vi "Process XML Node old2.vi"(8 "Error in":errorcluster caption="Error in (no error)", 11 "XML Element":refnum<k20>) -> (0 "Error out":errorcluster, 1 "Is Array?":bool, 2 "Attribute":refnum<class "Attribute.lvclass">, 3 "XML Element Out":refnum<k20>)   [LabVIEW 2018]
uses:
  Attribute.lvclass
  Data Item.lvclass/Data Item.ctl
  Element.lvclass/Element.ctl
  Element.lvclass
  C:/Users/Flarn/Documents/LabVIEW Projects/Low-Level VI Manipulation/Support Files/VILab/Data Item.lvclass
  Attribute.lvclass/Attribute.ctl
  Attribute/Create Attribute (Data Item).vi
  Element Array.lvclass
  Data Item.lvclass
  <vilib>/xml/NI_XML.lvlib
  <resource>/objmgr/DOMUserDefRef.rc
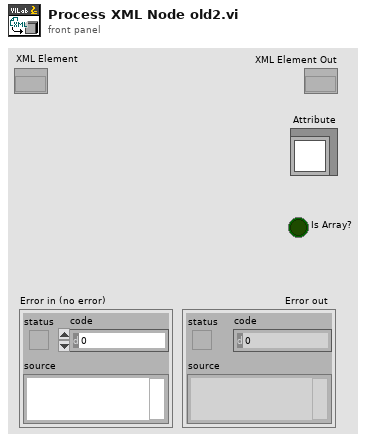
[diagram p1: front panel]
types:
  T1 = cluster{"class":string, "uid":string, "Attributes":refnum<class "Attribute.lvclass">[], "Array?":bool}
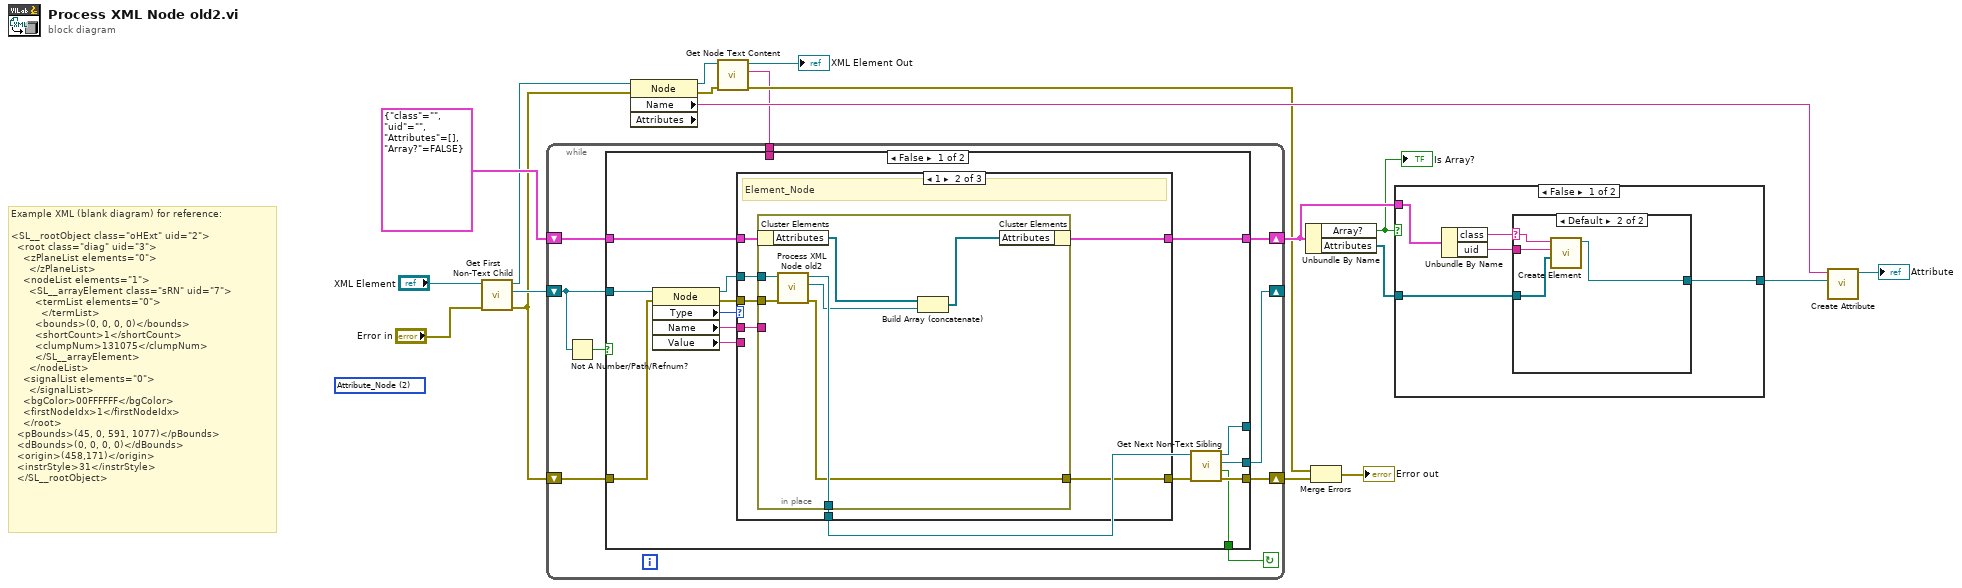
[diagram p0: block diagram]
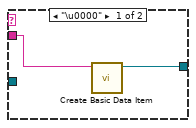
[diagram p2: hidden frame]
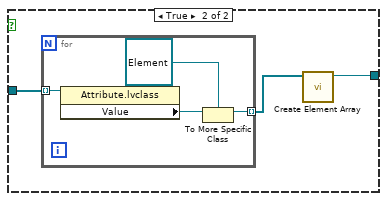
[diagram p3: hidden frame]
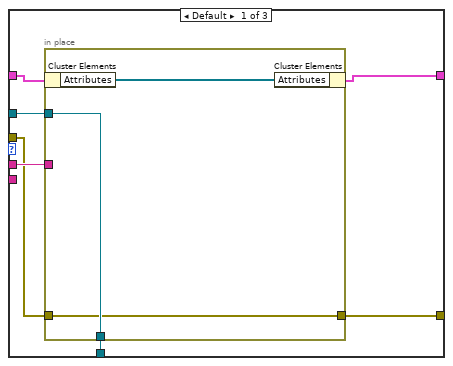
[diagram p4: hidden frame]
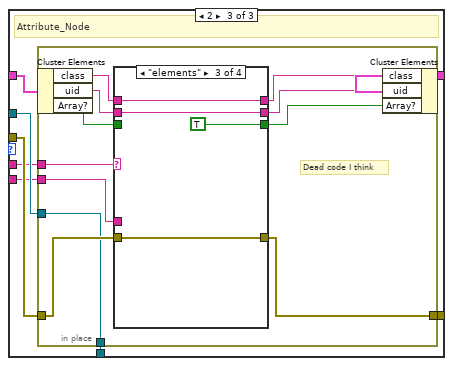
[diagram p5: hidden frame]
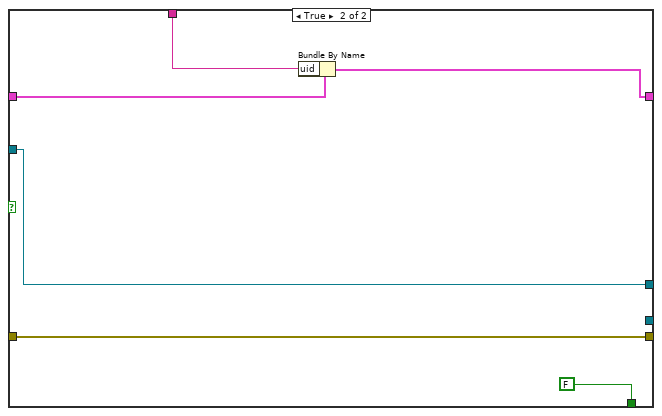
[diagram p9: hidden frame]
diagram:
  (unwired) 2 items=["Element_Node"=1, "Attribute_Node"=2, "Text_Node"=3, "CDATASection_Node"=4, "EntityReference_Node"=5, "Entity_Node"=6, "ProcessingInstruction_Node"=7, "Comment_Node"=8, "Document_Node"=9, "DocumentType_Node"=10, "DocumentFragment_Node"=11, "Notation_Node"=12] ("Node Type")
  # "Example XML (blank diagram) for reference:\n\n<SL__rootObject class=\"oHExt\" uid=\"2\">\n  <root class=\"diag\" uid=\"3\">\n    <zPlaneList elements=\"0\">\n      </zPlaneList>\n    <nodeList elements=\"1\">\n      <SL__arrayElement class=\"sRN\" uid=\"7\">\n        <termList elements=\"0\">\n          </termList>\n        <bounds>(0, 0, 0, 0)</bounds>\n        <shortCount>1</shortCount>\n        <clumpNum>131075</clumpNum>\n        </SL__arrayElement>\n      </nodeList>\n    <signalList elements=\"0\">\n      </signalList>\n    <bgColor>00FFFFFF</bgColor>\n    <firstNodeIdx>1</firstNodeIdx>\n    </root>\n  <pBounds>(45, 0, 591, 1077)</pBounds>\n  <dBounds>(0, 0, 0, 0)</dBounds>\n  <origin>(458,171)</origin>\n  <instrStyle>31</instrStyle>\n  </SL__rootObject>"
  n1 = call <vilib>:"Get First Non-Text Child.vi"("error in (no error)"="Error in", "node in"="XML Element") -> ("error out"=w6:errorcluster, "child node"=w18:refnum<k20>, "node out"=w12:refnum<k20>)  [unwired: 6 in, 1 out]
  n2 = property class="Node" props=["Name", "Attributes"](reference=w12, error in=w6) -> (reference out=w8:refnum<k20>, error out=w5:errorcluster, "Name"=w10:string)  [unwired: 1 out]
  n3 = call <vilib>:"Get Node Text Content.vi"("error in (no error)"=w5, "node in"=w8) -> ("error out"=w4:errorcluster, "node text"=w1:string, "node out"=→"XML Element Out":refnum<k20>)  [unwired: 7 in]
  n4 = while {
    shift-right: [w24] -> w14
    shift-left: T1 {"class"="", "uid"="", "Attributes"=[], "Array?"=FALSE} -> [w25]
    shift-right: [w28] -> w3
    shift-left: w6 -> [w26]
    shift-right: [w23] -> _
    shift-left: w18 -> [w21]
    tunnel: w1 -> [w20]
    stop <- w27 continue-if-true
    n5 = Not A Number/Path/Refnum?(number/path/refnum=w21) -> (NaN/Path/Refnum?=w22:bool)
    n6 = case shown="False" w22 {
      tunnel: [w43 w108] -> w28
      tunnel: [w42 FALSE ("found sibling node?")] -> w27
      tunnel: w21 -> [w41 w106]
      tunnel: w26 -> [w39 w108]
      tunnel: w25 -> [w36 w105]
      tunnel: [w35 w103] -> w24
      tunnel: [w33 _] -> w23
      tunnel: [w31 w106] -> _
      tunnel: w20 -> [_ w104]
      frame False {
        n7 = property class="Node"(reference=w41, error in=w39) -> (reference out=w37:refnum<k20>, error out=w38:errorcluster, "Type"=w40:i32, "Name"=w30:string, "Value"=w29:string)
        n8 = case shown="1" w40 {
          tunnel: w38 -> [w45 w60 w75]
          tunnel: w37 -> [w49 w59 w72]
          tunnel: w36 -> [w47 w58 w73]
          tunnel: [w46 w57 w74] -> w35
          tunnel: [w44 w56 w71] -> w34
          tunnel: [w50 w55 w70] -> w32
          tunnel: w30 -> [w48 w54 w69]
          tunnel: w29 -> [_ _ w68]
          frame Default {
            n9 = in-place {
              in-place-border: [w53] -> w50
              in-place-border: w49 -> [w53]
              in-place-border: w48 -> [_]
              in-place-border: w45 -> [w52]
              in-place-border: [w52] -> w44
              n10 = in-place-cluster #1(w47) -> ("Attributes"=w51:refnum<class "Attribute.lvclass">[])
              n11 = in-place-cluster #1("Attributes"=w51) -> (w46:T1)
            }
          }
          frame 1 {
            # "Element_Node"
            n12 = in-place {
              in-place-border: w60 -> [w67]
              in-place-border: w59 -> [w66]
              in-place-border: [w61] -> w56
              in-place-border: [w63] -> w55
              in-place-border: w54 -> [_]
              n13 = in-place-cluster #2(w58) -> ("Attributes"=w65:refnum<class "Attribute.lvclass">[])
              n14 = call "Process XML Node old2.vi"("Error in"=w67, "XML Element"=w66) -> ("Error out"=w61:errorcluster, "Attribute"=w62:refnum<class "Attribute.lvclass">, "XML Element Out"=w63:refnum<k20>)  [unwired: 6 in, 1 out]
              n15 = Build Array (concatenate)(w65, w62) -> (w64:refnum<class "Attribute.lvclass">[])
              n16 = in-place-cluster #2("Attributes"=w64) -> (w57:T1)
            }
          }
          frame 2 {
            # "Attribute_Node"
            n17 = in-place {
              in-place-border: w75 -> [w79]
              in-place-border: w69 -> [w86]
              in-place-border: w72 -> [w77]
              in-place-border: [w78] -> w71
              in-place-border: [w77] -> w70
              in-place-border: w68 -> [w76]
              # "Dead code I think"
              n18 = in-place-cluster #3(w73) -> ("class"=w85:string, "uid"=w84:string, "Array?"=w83:bool)
              n19 = case shown="\"elements\"" w86 {
                tunnel: w85 -> [_ w94 w98 w102]
                tunnel: w84 -> [w90 _ w97 w101]
                tunnel: w83 -> [w89 w93 _ w100]
                tunnel: [w87 w94 w98 w102] -> w82
                tunnel: [w90 w91 w97 w101] -> w81
                tunnel: [w89 w93 TRUE w100] -> w80
                tunnel: w79 -> [w88 w92 w96 w99]
                tunnel: [w88 w92 w96 w99] -> w78
                tunnel: w76 -> [w87 w91 _ _]
                frame "class" {
                }
                frame "uid" {
                }
                frame "elements" {
                }
                frame Default {
                }
              }
              n20 = in-place-cluster #3("class"=w82, "uid"=w81, "Array?"=w80) -> (w74:T1)
            }
          }
        }
        n21 = call <vilib>:"Get Next Non-Text Sibling.vi"("error in (no error)"=w34, "node in"=w32) -> ("error out"=w43:errorcluster, "found sibling node?"=w42:bool, "sibling node"=w33:refnum<k20>, "node out"=w31:refnum<k20>)  [unwired: 6 in]
      }
      frame True {
        n22 = Bundle By Name(cluster=w105, "uid"=w104) -> (w103:T1)
      }
    }
  }
  n23 = Unbundle By Name(w14) -> ("Array?"=w13:bool, "Attributes"=w15:refnum<class "Attribute.lvclass">[])
  "Is Array?" <- w13
  n24 = Merge Errors(w4, w3) -> (→"Error out":errorcluster)
  n25 = case shown="False" w13 {
    tunnel: w15 -> [w111 w122]
    tunnel: [w110 w120] -> w11
    tunnel: w14 -> [w113 _]
    frame False {
      n26 = Unbundle By Name(w113) -> ("class"=w109:string, "uid"=w112:string)
      n27 = case shown="Default" w109 {
        selector: w109 -> [_ w116]
        tunnel: w112 -> [w115 w119]
        tunnel: w111 -> [_ w118]
        tunnel: [w114 w117] -> w110
        frame "\u0000" {
          n28 = call "Create Basic Data Item.vi"("Content"=w115) -> ("New Data Item"=w114:refnum<class "Data Item.lvclass">)  [unwired: 10 in]
        }
        frame Default {
          n29 = call "Create Element.vi"("Attributes"=w118, "uid"=w119, "class"=w116) -> ("Element"=w117:refnum<class "Element.lvclass">)  [unwired: 8 in]
        }
      }
    }
    frame True {
      n30 = for {
        tunnel: w122 -> [w126] mode=indexing
        tunnel: [w123] -> w121 mode=indexing
        n31 = property class="Attribute.lvclass"(reference=w126) -> ("Value"=w125:refnum<class "Data Item.lvclass">)  [unwired: 1 in, 2 out]
        n32 = To More Specific Class(target class=refnum<class "Element.lvclass"> refnum ("VILab.lvlib:Element.lvclass"), reference=w125) -> (specific class reference=w123:refnum<class "Element.lvclass">)  [unwired: 1 in, 1 out]
      }
      n33 = call "Create Element Array.vi"("Contents"=w121) -> ("Element Array"=w120:refnum<class "Element Array.lvclass">)  [unwired: 9 in, 1 out]
    }
  }
  n34 = call-poly "Create Attribute.vi"("Value"=w11, "Name"=w10) -> ("Attribute"=→"Attribute":refnum<class "Attribute.lvclass">)  [unwired: 9 in]
